vi "Close.vi"(8 "error in (no error)":errorcluster, 9 "ms Timeout (2000)":u32=2000, 11 "App ID in":u16) -> (0 "error out":errorcluster)   [LabVIEW 2018, in "TCPServer.lvlib"]
uses:
  TCPServer.lvlib
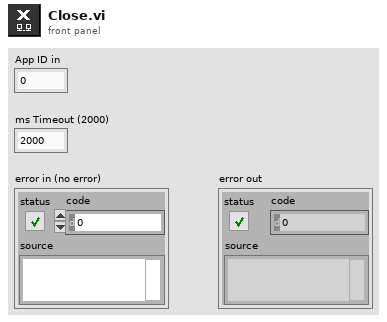
[diagram p1: front panel]
types:
  T1 = typedef "TCPServer.lvlib/App.ctl" = cluster{"Stack":refnum<queue>, "Cmd":cluster{"Conn":refnum<data-value>, "Daemon":refnum<vi>, "Counter":refnum<data-value>}, "Tlm":cluster{"Conn":refnum<data-value>, "Daemon":refnum<vi>, "Counter":refnum<data-value>}}
  T2 = cluster{"Conn":refnum<data-value>, "Daemon":refnum<vi>, "Counter":refnum<data-value>}
  T3 = cluster{"Conn":refnum<data-value>, "Daemon":refnum<vi>, "Counter":refnum<data-value>}[]
  T4 = typedef "TCPServer.lvlib/Connection.ctl" = cluster{"Tcp":refnum<k5>, "Server Port":u16, "Server Port Type":enum8{"CMD", "TLM", "BOTH"}, "Client IP":string, "Client Port":u16}
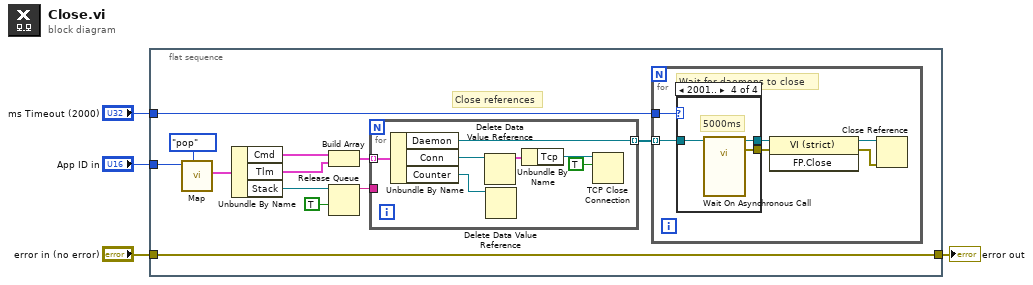
[diagram p0: block diagram]
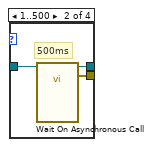
[diagram p3: hidden frame]
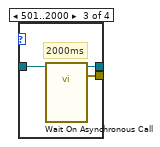
[diagram p4: hidden frame]
diagram:
  n1 = flat-sequence {
    tunnel: "App ID in" -> [w16]
    tunnel: "ms Timeout (2000)" -> [w14]
    tunnel: [w6] -> w2
    tunnel: "error in (no error)" -> [w6]
    frame #0 {
      # "Close references"
      n2 = call "Map.vi"("Action"=enum8{"noop", "get", "set", "pop"}."pop", "App ID in"=w16) -> ("App out"=w11:T1)  [unwired: 7 in, 2 out]
      n3 = Unbundle By Name(w11) -> ("Cmd"=w10:T2, "Tlm"=w9:T2, "Stack"=w7:refnum<queue>)
      n4 = Build Array(w10, w9) -> (w8:T3)
      n5 = Release Queue(queue=w7, force destroy? (F)=TRUE) -> (queue name=w5:string)  [unwired: 1 in, 2 out]
      n6 = for {
        tunnel: w8 -> [w38] mode=indexing
        tunnel: [w33] -> w15 mode=indexing
        tunnel: w5 -> [_]
        n7 = Unbundle By Name(w38) -> ("Daemon"=w33:refnum<vi>, "Conn"=w35:refnum<data-value>, "Counter"=w34:refnum<data-value>)
        n8 = Delete Data Value Reference(data value reference=w35) -> (data value=w37:T4)  [unwired: 1 in, 1 out]
        n9 = Delete Data Value Reference(data value reference=w34) -> ()  [unwired: 1 in, 2 out]
        n10 = Unbundle By Name(w37) -> ("Tcp"=w39:refnum<k5>)
        n11 = TCP Close Connection(connection ID=w39, abort (F)=TRUE) -> ()  [unwired: 1 in, 2 out]
      }
      n12 = for {
        tunnel: w15 -> [w17] mode=indexing
        tunnel: w14 -> [w18]
        # "Wait for daemons to close"
        n13 = case shown="2001.." w18 {
          tunnel: w17 -> [w23 w26 w29 w32]
          tunnel: [_ w25 w28 w31] -> w22
          tunnel: [w23 w24 w27 w30] -> w21
          frame 0 {
          }
          frame 1..500 {
            # "500ms"
            n14 = call-by-ref "Wait On Asynchronous Call"(reference=w26) -> (reference out=w24:refnum<vi>, error out=w25:errorcluster)  [unwired: 13 in]
          }
          frame 501..2000 {
            # "2000ms"
            n15 = call-by-ref "Wait On Asynchronous Call"(reference=w29) -> (reference out=w27:refnum<vi>, error out=w28:errorcluster)  [unwired: 13 in]
          }
          frame 2001.. {
            # "5000ms"
            n16 = call-by-ref "Wait On Asynchronous Call"(reference=w32) -> (reference out=w30:refnum<vi>, error out=w31:errorcluster)  [unwired: 13 in]
          }
        }
        n17 = invoke class="VI (strict)" method="FP.Close"(reference=w21, error in=w22) -> (reference out=w20:refnum<vi>, error out=w19:errorcluster)  [unwired: 1 in, 1 out]
        n18 = Close Reference(reference=w20, error in (no error)=w19) -> ()  [unwired: 1 out]
      }
    }
  }
  "error out" <- w2
